vi "Main.vi"() -> ()   [LabVIEW 2012]
doc: "Use this template to build a simple state machine design pattern. Each state executes code and determines which state to transition to."
uses:
  controls/Data.ctl
  <vilib>/express/express shared/transition.llb/Dynamic To Waveform Array.vi
  <vilib>/express/express shared/transition.llb/Waveform Array To Dynamic.vi
  <vilib>/express/express arith-compare/Formula/Block/exnFormulaBlock how many pts in the wave.vi
  <vilib>/express/express shared/ex_Modify Signal Name.vi
  <vilib>/express/express arith-compare/Formula/XNode/ExpressFormulaBlockNode.xnode
panel:
  out "Elapsed time (sec)":dbl format="%#.3f"
  out "RecCount":i32
  in  "Period (sec)":dbl=3.0
  out "Coated Temperature":dbl
  out "Bare Temperature":dbl
  out "Low Airflow":bool
  out "PWM On":bool
  in  "Stop":bool=TRUE
  in  "Filename to save to":path=path "Z:/adit/Desktop/MEL III/RefrigerationData.lvm" caption="Filename"
  in  "Save Data?":bool=TRUE
  out "Derivative Output":dbl
  out "Integral Output":dbl
  out "CO Bias":dbl
  out "Proportional Output":dbl
  out "Duty Cycle":dbl
  out "Current Set Point":dbl
  out "Flow Rate":dbl
  in  "Integral Constant":dbl=0.1 caption="I Coefficient" format="%0.2f"
  in  "Derivative \nConstant":dbl=0.05 caption="D Coefficient" format="%0.2f"
  in  "Proportional\nConstant":dbl=1.0 caption="P Coefficient" format="%0.2f"
  in  "Duty Cycle\nincrement amount":dbl=1.0
  in  "Decrease Duty Cycle":bool
  in  "Increase Duty Cycle":bool
  in  "Set Point\nIncrement amount":dbl=1.0
  in  "Lower Set Point":bool
  in  "Raise Set Point":bool
  in  "Bare(T) or \nCoated?":bool
  in  "Manual / Auto":bool
  in  "Time to wait(ms)":u32
  in  "Readings between\nrecorded data":i32
  out "Bare Temperature":dbl
  out "Coated Temperature":dbl
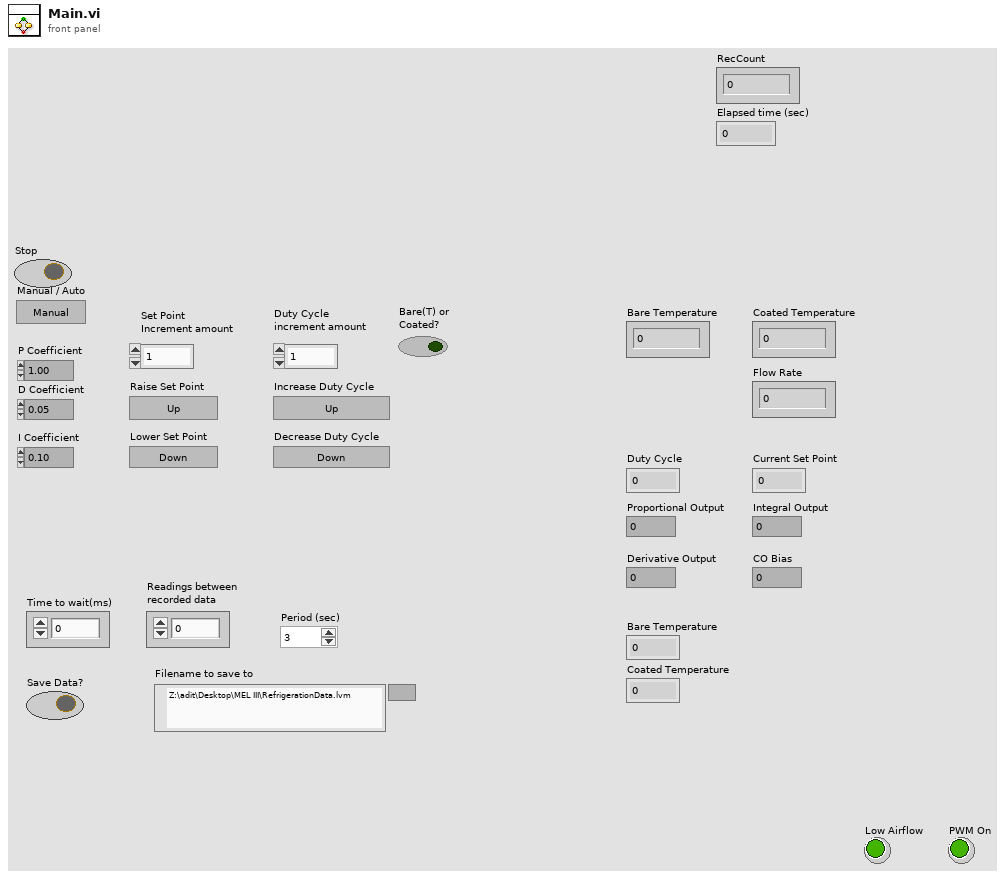
[diagram p1: front panel]
types:
  T1 = cluster{"RecCount":i32, "Starting Tick Count":i32, "Coated Probe":dbl, "Uncoated Probe":dbl, "Mass Flow":dbl, "Derivative Out":dbl, "Integral Out":dbl, "Proportional Out":dbl, "Manual/Auto":bool, "Set Point":dbl, "Duty Cycle":dbl, "Pwm Value":dbl}
  T2 = enum16{"Initialize", "Acquire", "Analyze", "PID", "Record", "PWM", "Output", ""}
  T3 = typedef "Data.ctl" = cluster{"Boolean <Replace Me>":bool, "String <Replace Me>":string, "Numeric <Replace Me>":dbl}
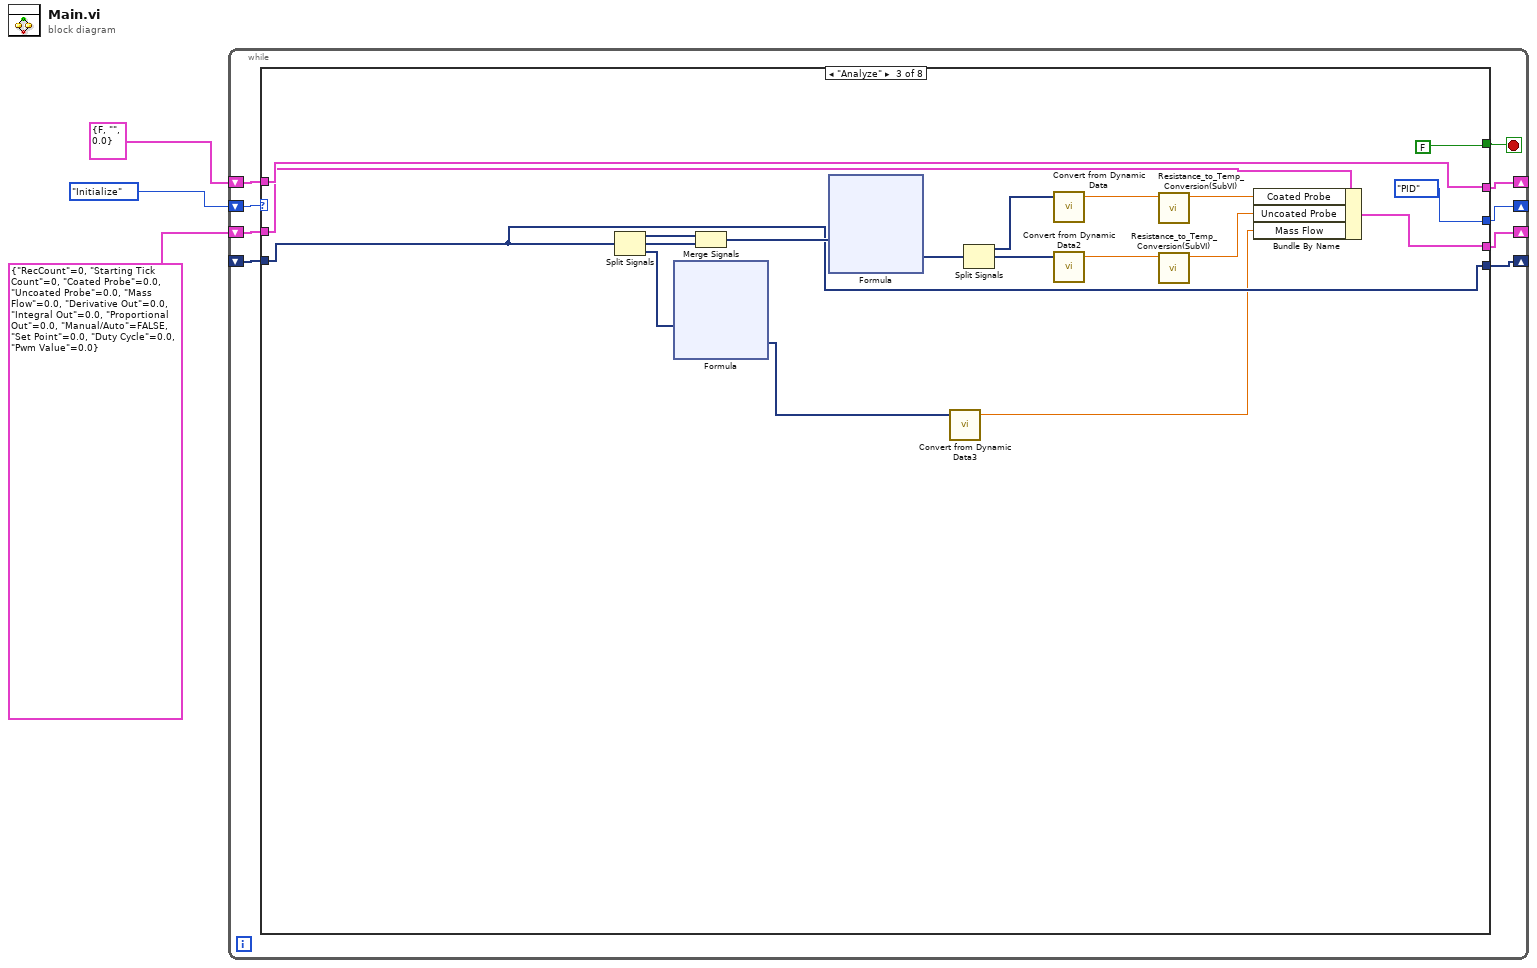
[diagram p0: block diagram]
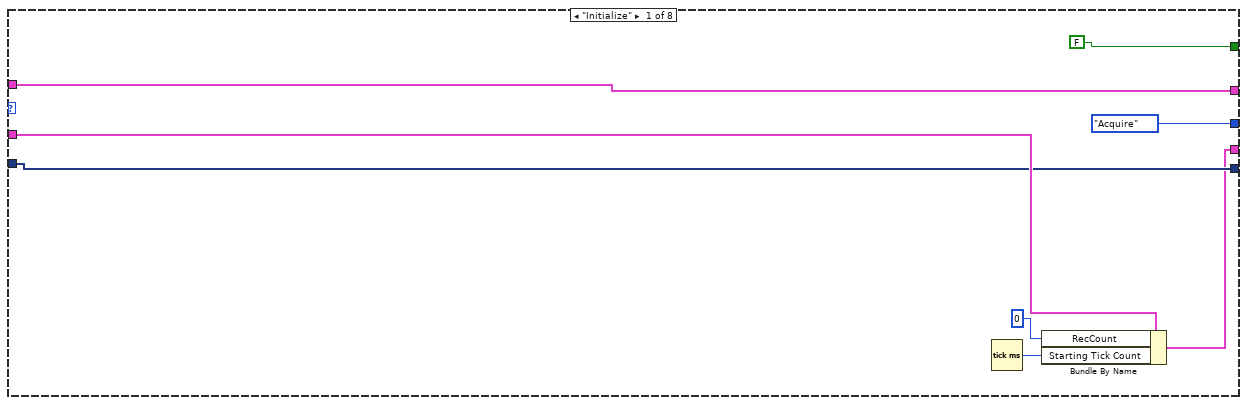
[diagram p2: hidden frame]
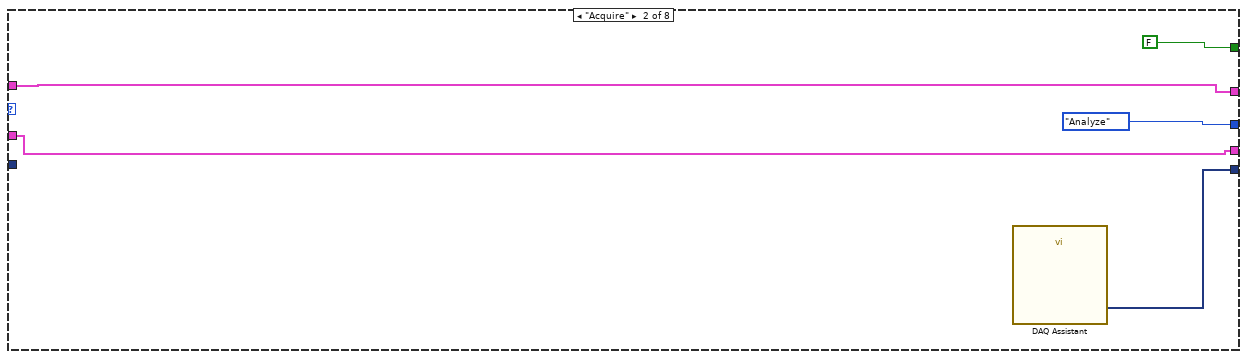
[diagram p3: hidden frame]
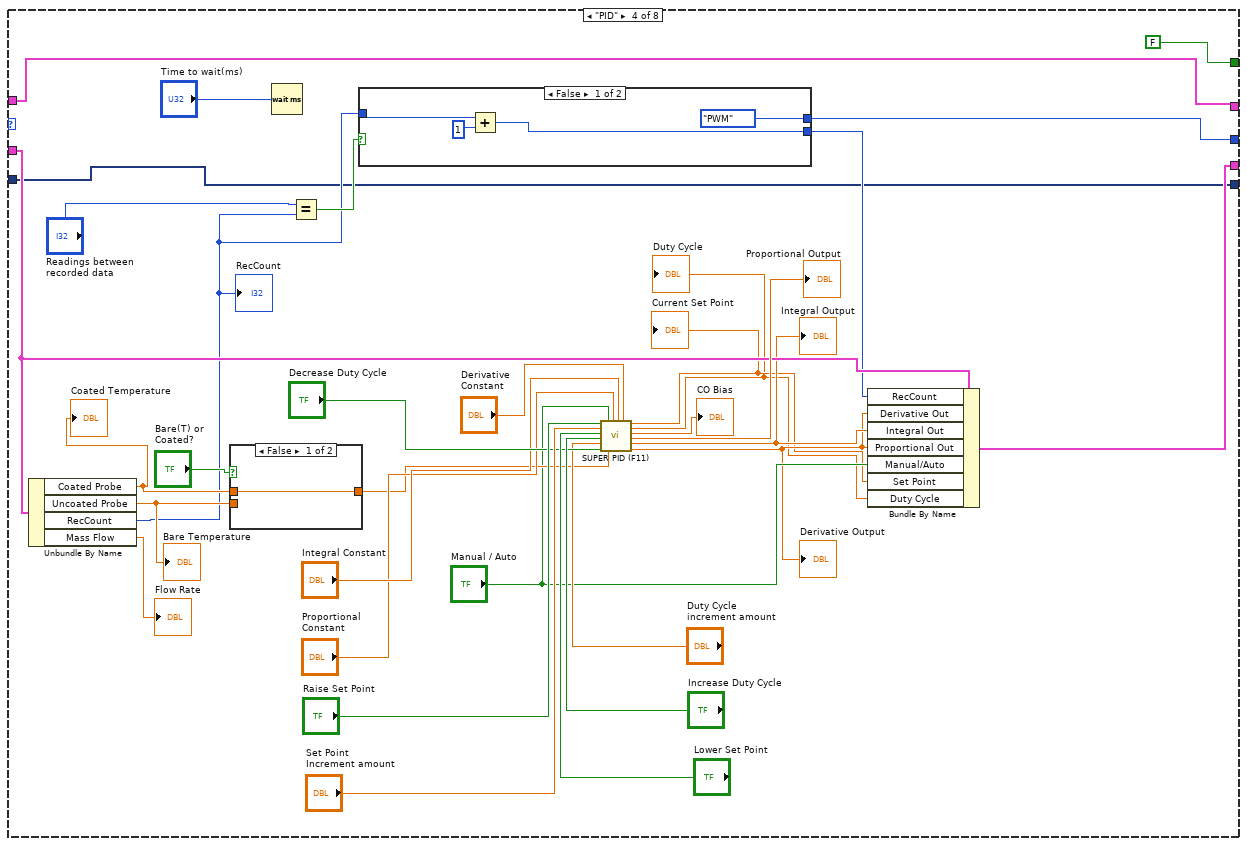
[diagram p4: hidden frame]
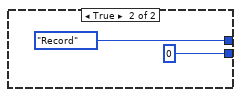
[diagram p6: hidden frame]
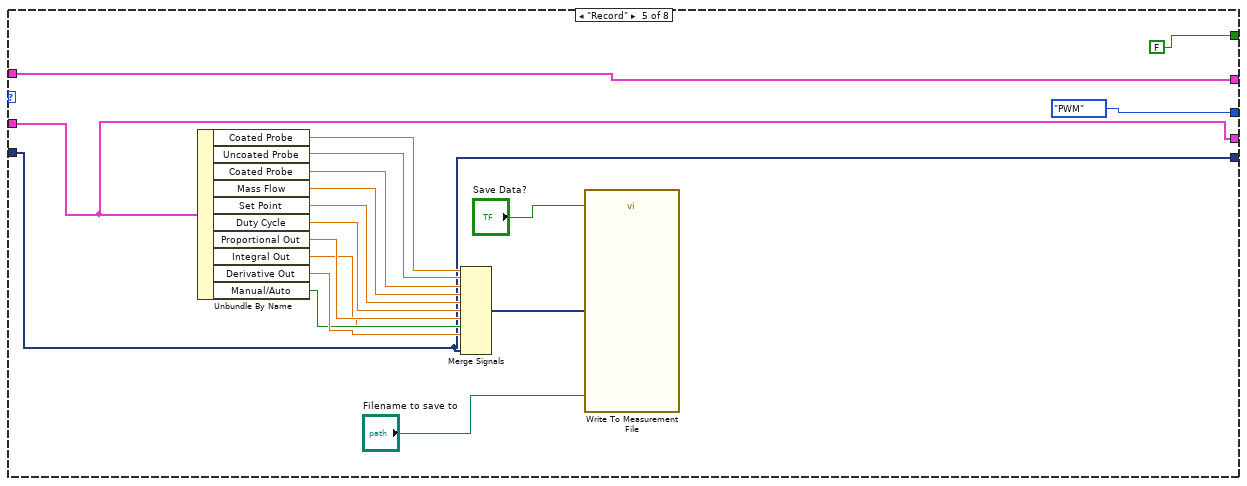
[diagram p7: hidden frame]
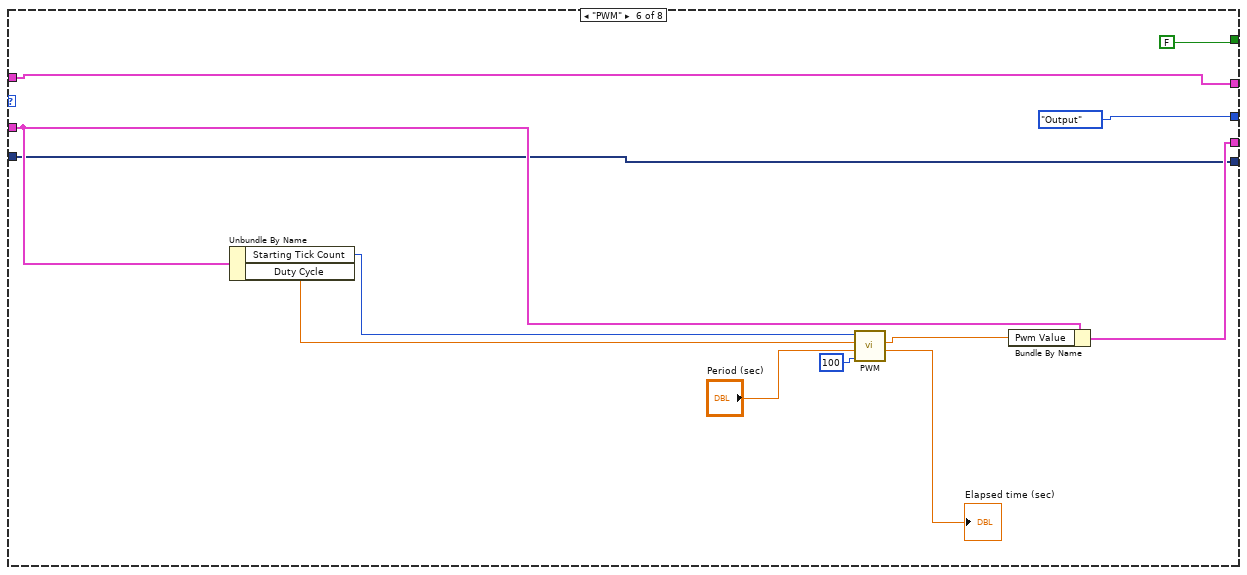
[diagram p8: hidden frame]
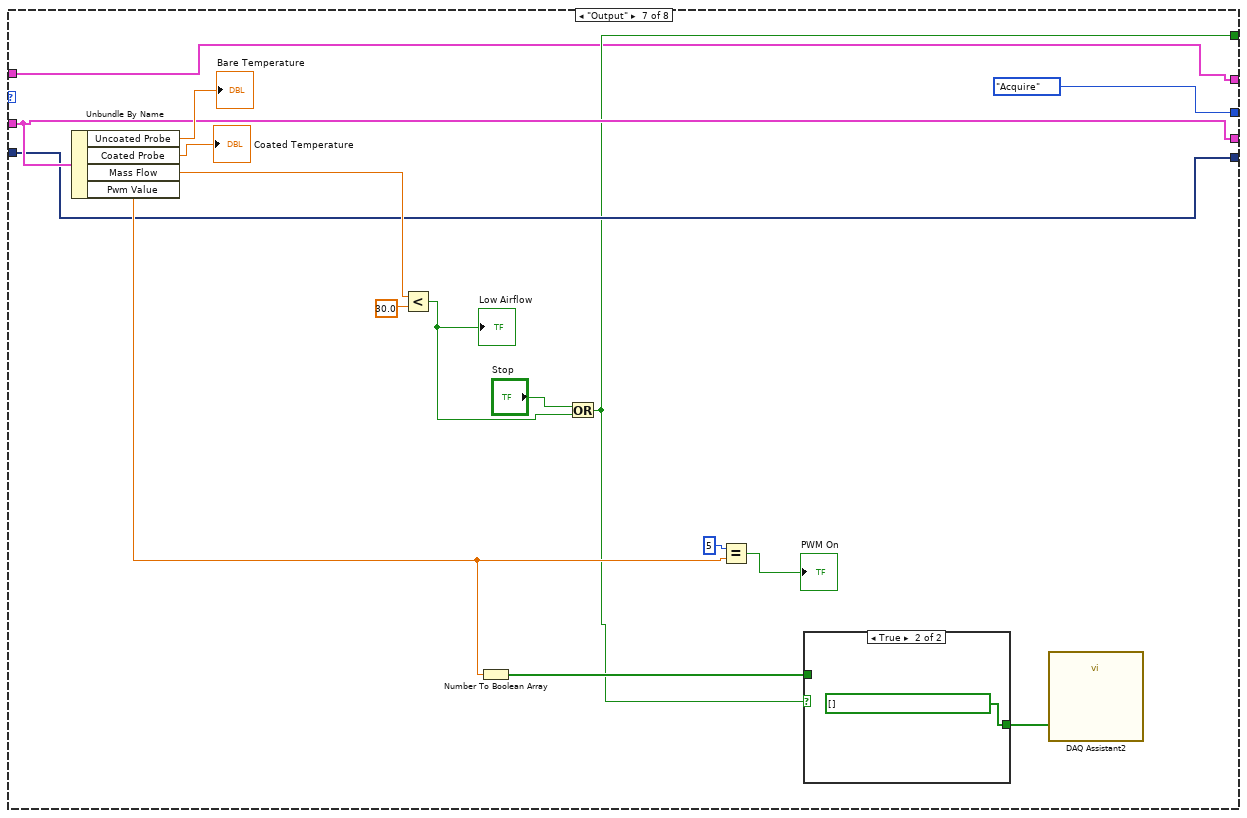
[diagram p9: hidden frame]
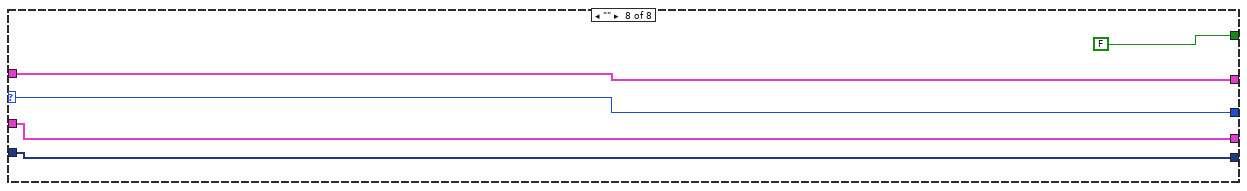
[diagram p11: hidden frame]
diagram:
  n1 = while {
    shift-right: [w11] -> _
    shift-left: T2."Initialize" -> [w12]
    shift-right: [w9] -> _
    shift-left: T3 {"Boolean <Replace Me>"=FALSE, "String <Replace Me>"="", "Numeric <Replace Me>"=0.0} ("Data") -> [w10]
    shift-right: [w6] -> _
    shift-left: T1 {"RecCount"=0, "Starting Tick Count"=0, "Coated Probe"=0.0, "Uncoated Probe"=0.0, "Mass Flow"=0.0, "Derivative Out"=0.0, "Integral Out"=0.0, "Proportional Out"=0.0, "Manual/Auto"=FALSE, "Set Point"=0.0, "Duty Cycle"=0.0, "Pwm Value"=0.0} -> [w7]
    shift-right: [w5] -> _
    shift-left: _ -> [w4]
    stop <- w8 stop-if-true
    n2 = case shown="\"Analyze\"" w12 {
      selector: w12 -> [_ _ _ _ _ _ _ w414]
      tunnel: [T2."Acquire" T2."Analyze" T2."PID" w341 T2."PWM" T2."Output" T2."Acquire" w414] -> w11
      tunnel: [FALSE FALSE FALSE ("Stop Loop?") FALSE ("Stop Loop?") FALSE FALSE w394 FALSE ("Stop Loop?")] -> w8
      tunnel: w10 -> [w20 w24 w44 w323 w380 w392 w393 w415]
      tunnel: [w20 w24 w44 w323 w380 w392 w393 w415] -> w9
      tunnel: [w16 w22 w29 w324 w364 w382 w395 w411] -> w5
      tunnel: w7 -> [w19 w21 w33 w335 w365 w386 w396 w412]
      tunnel: [w15 w21 w28 w325 w365 w384 w396 w412] -> w6
      tunnel: w4 -> [w16 _ w29 w324 w364 w382 w395 w411]
      frame "Initialize" {
        n3 = Tick Count (ms)() -> (millisecond timer value=w17:u32)
        n4 = Bundle By Name(cluster=w19, "RecCount"=0, "Starting Tick Count"=w17) -> (w15:T1)
      }
      frame "Acquire" {
        n5 = call "DAQ Assistant"() -> ("data"=w22:dynamicdata)  [unwired: 17 in, 2 out]
      }
      frame "Analyze" {
        n6 = Split Signals(w29) -> (w36:dynamicdata, w34:dynamicdata, w35:dynamicdata)  [unwired: 3 in]
        n7 = xnode "Formula"("V"=w35) -> ("Result"=w27:dynamicdata)  [unwired: 1 in, 1 out]
        n8 = Merge Signals(w36, w34) -> (w37:dynamicdata)
        n9 = xnode "Formula"("V"=w37) -> ("Result"=w42:dynamicdata)  [unwired: 1 in, 1 out]
        n10 = call "Convert from Dynamic Data3"("Dynamic Data Type"=w27) -> ("Scalar"=w26:dbl)  [unwired: 3 in]
        n11 = Split Signals(w42) -> (w41:dynamicdata, w40:dynamicdata)  [unwired: 3 in, 1 out]
        n12 = call "Convert from Dynamic Data"("Dynamic Data Type"=w41) -> ("Scalar"=w38:dbl)  [unwired: 3 in]
        n13 = call "Convert from Dynamic Data2"("Dynamic Data Type"=w40) -> ("Scalar"=w39:dbl)  [unwired: 3 in]
        n14 = call "Resistance_to_Temp_Conversion(SubVI).vi"("Scalar"=w38) -> ("Result"=w32:dbl)  [unwired: 10 in]
        n15 = call "Resistance_to_Temp_Conversion(SubVI).vi"("Scalar"=w39) -> ("Result"=w31:dbl)  [unwired: 10 in]
        n16 = Bundle By Name(cluster=w33, "Coated Probe"=w32, "Uncoated Probe"=w31, "Mass Flow"=w26) -> (w28:T1)
      }
      frame "PID" {
        n17 = Unbundle By Name(w335) -> ("Coated Probe"=w327:dbl, "Uncoated Probe"=w336:dbl, "RecCount"=w326:i32, "Mass Flow"=→"Flow Rate":dbl)
        "Coated Temperature" <- w327
        "Bare Temperature" <- w336
        "RecCount" <- w326
        n18 = case shown="False" "Bare(T) or \nCoated?" {
          tunnel: w327 -> [w355 _]
          tunnel: w336 -> [_ w356]
          tunnel: [w355 w356] -> w337
          frame False {
          }
          frame True {
          }
        }
        n19 = Wait (ms)(milliseconds to wait="Time to wait(ms)") -> ()  [unwired: 1 out]
        n20 = Equal?(x="Readings between\nrecorded data", y=w326) -> (x = y?=w344:bool)
        n21 = case shown="False" w344 {
          tunnel: [T2."PWM" T2."Record"] -> w341
          tunnel: [w358 0] -> w334
          tunnel: w326 -> [w357 _]
          frame False {
            n22 = Add(x=w357, y=1) -> (x+y=w358:i32)
          }
          frame True {
          }
        }
        n23 = call "SUPER PID (F11).vi"("SP Up"="Raise Set Point", "SP Increment"="Set Point\nIncrement amount", "SP Down"="Lower Set Point", "DC Up"="Increase Duty Cycle", "DC Increment"="Duty Cycle\nincrement amount", "DC Down"="Decrease Duty Cycle", "Manual / Auto"="Manual / Auto", "PV"=w337, "P"="Proportional\nConstant", "I"="Integral Constant", "D"="Derivative \nConstant") -> ("SP"=w330:dbl, "DC"=w329:dbl, "CO Bias"=→"CO Bias":dbl, "P out"=→"Proportional Output":dbl, "I out"=w333:dbl, "D out"=w331:dbl)  [unwired: 3 in]
        "Current Set Point" <- w330
        "Duty Cycle" <- w329
        "Integral Output" <- w333
        "Derivative Output" <- w331
        n24 = Bundle By Name(cluster=w335, "RecCount"=w334, "Derivative Out"=w331, "Integral Out"=w333, "Proportional Out"=w331, "Manual/Auto"="Manual / Auto", "Set Point"=w330, "Duty Cycle"=w329) -> (w325:T1)
      }
      frame "Record" {
        n25 = Unbundle By Name(w365) -> ("Coated Probe"=w375:dbl, "Uncoated Probe"=w374:dbl, "Coated Probe"=w373:dbl, "Mass Flow"=w372:dbl, "Set Point"=w371:dbl, "Duty Cycle"=w370:dbl, "Proportional Out"=w369:dbl, "Integral Out"=w366:dbl, "Derivative Out"=w368:dbl, "Manual/Auto"=w367:bool)
        n26 = Merge Signals(w375, w374, w373, w372, w371, w370, w369, w366, w368, w367, w364) -> (w376:dynamicdata)
        n27 = call "Write To Measurement File"("Signals"=w376, "Reset"="Save Data?", "Filename"="Filename to save to") -> ()  [unwired: 14 in, 3 out]
      }
      frame "PWM" {
        n28 = Unbundle By Name(w386) -> ("Starting Tick Count"=w388:i32, "Duty Cycle"=w387:dbl)
        n29 = call "PWM.vi"("milliseconds to wait 2"=u32 100 ("milliseconds to wait"), "Period (sec) 2"="Period (sec)", "Duty Cycle 2"=w387, "Starting tic count"=w388) -> ("Elapsed time (sec) 2"=→"Elapsed time (sec)":dbl, "Pwm output 2"=w385:dbl)  [unwired: 6 in]
        n30 = Bundle By Name(cluster=w386, "Pwm Value"=w385) -> (w384:T1)
      }
      frame "Output" {
        n31 = Unbundle By Name(w396) -> ("Uncoated Probe"=→"Bare Temperature":dbl, "Coated Probe"=→"Coated Temperature":dbl, "Mass Flow"=w400:dbl, "Pwm Value"=w399:dbl)
        n32 = Less?(x=w400, y=30.0) -> (x < y?=w403:bool)
        "Low Airflow" <- w403
        n33 = Number To Boolean Array(number=w399) -> (Boolean array=w398:bool[])
        n34 = Or(x="Stop", y=w403) -> (x .or. y?=w394:bool)
        n35 = Equal?(x=5, y=w399) -> (x = y?=→"PWM On":bool)
        n36 = case shown="True" w394 {
          tunnel: w398 -> [w409 _]
          tunnel: [w409 bool[] []] -> w397
          frame False {
          }
          frame True {
          }
        }
        n37 = call "DAQ Assistant2"("data"=w397) -> ()  [unwired: 17 in, 2 out]
      }
      frame "" {
      }
    }
  }
